vi "Begin.vi"(8 "error in (no error)":errorcluster, 11 "DriveMotorsLeft in":refnum<class "DriveMotorsLeft.lvclass">) -> (0 "error out":errorcluster, 3 "DriveMotorsLeft out":refnum<class "DriveMotorsLeft.lvclass">)   [LabVIEW 2013, in "DriveMotorsLeft.lvclass"]
uses:
  DriveMotorsLeft.lvclass
  DriveMotors/DriveMotors.lvclass
  <vilib>/Rock Robotics/WPI/MotorControl/WPI_MotorControlOpenCANJaguar.vi
panel:
  in  "Motor3Can 2":u8=16
  in  "Motor2Can":u8=15
  in  "Motor1CAN":u8=14
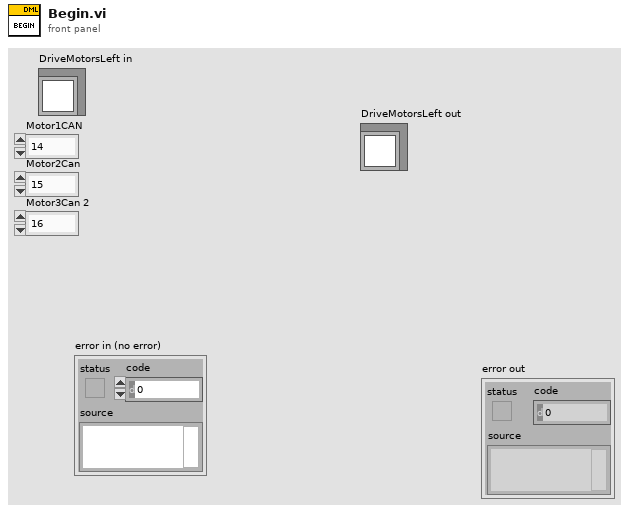
[diagram p1: front panel]
types:
  T1 = typedef "WPI_MotorControlDeviceRef.ctl" = cluster{"DeviceStatus":errorcluster, "Type":enum16{"PWM", "CAN"}, "PWM":cluster{"Digital Module":T2, "PWM Channel":T3, "DeadBand":T4}, "CAN":cluster{"Device Number":u8, "Control Mode":T5, "Semaphore":T6, "Max Vout":dbl}, "Invert":bool, "TransformRef":T7, "InvTransformRef":T7}
  T2 = typedef "FPGA_TypedefDigitalModule.ctl" = enum16{"Digital Module 1", "Digital Module 2"}
  T3 = typedef "FPGA_DIOPWMChannel.ctl" = enum8{"PWM 1", "PWM 2", "PWM 3", "PWM 4", "PWM 5", "PWM 6", "PWM 7", "PWM 8", "PWM 9", "PWM 10", "Invalid"}
  T4 = typedef "WPI_PWMDeadband.ctl" = cluster{"Name":string, "maxPositivePwm":i32, "minPositivePwm":i32, "centerPwm":i32, "maxNegativePwm":i32, "minNegativePwm":i32, "angularRange":u16}
  T5 = typedef "WPI_CANJaguar_ControlMode.ctl" = enum8{"Percent VBus", "Current", "Speed", "Position", "Voltage"}
  T6 = typedef "Semaphore RefNum" = refnum<k1>
  T7 = typedef "WPI_PWMTransform_ConPane.ctl" = refnum<vi>
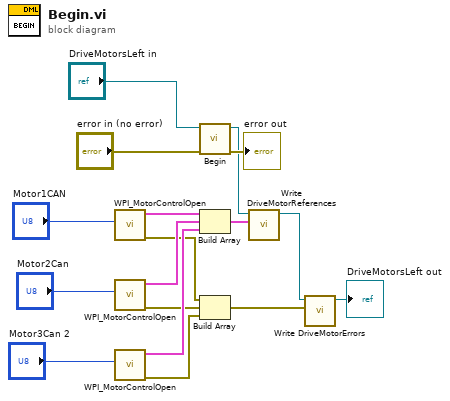
[diagram p0: block diagram]
diagram:
  n1 = call-poly <vilib>:"WPI_MotorControlOpen.vi"("Device Number"="Motor1CAN") -> ("error out"=w6:errorcluster, "MotorControlDeviceRef"=w10:T1)  [unwired: 9 in]
  n2 = call-poly <vilib>:"WPI_MotorControlOpen.vi"("Device Number"="Motor2Can") -> ("error out"=w5:errorcluster, "MotorControlDeviceRef"=w9:T1)  [unwired: 9 in]
  n3 = call-poly <vilib>:"WPI_MotorControlOpen.vi"("Device Number"="Motor3Can 2") -> ("error out"=w4:errorcluster, "MotorControlDeviceRef"=w8:T1)  [unwired: 9 in]
  n4 = call-parent "Begin.vi"("error in (no error)"="error in (no error)", "DriveMotors in"="DriveMotorsLeft in") -> ("error out"=→"error out":errorcluster, "DriveMotors out"=w11:refnum<class "DriveMotorsLeft.lvclass">)  [unwired: 8 in]
  n5 = Build Array(w10, w9, w8) -> (w7:T1[])
  n6 = Build Array(w6, w5, w4) -> (w1:errorcluster[])
  n7 = call-dynamic "Write DriveMotorReferences.vi"("DriveMotorReferences"=w7, "DriveMotors in"=w11) -> ("DriveMotors out"=w3:refnum<class "DriveMotorsLeft.lvclass">)  [unwired: 8 in, 1 out]
  n8 = call-dynamic "Write DriveMotorErrors.vi"("DriveMotorErrors"=w1, "DriveMotors in"=w3) -> ("DriveMotors out"=→"DriveMotorsLeft out":refnum<class "DriveMotorsLeft.lvclass">)  [unwired: 8 in, 1 out]
